vi "Post-Install Custom Action.vi"(10 "Variant":variant) -> (0 "error out":errorcluster)   [LabVIEW 2014]
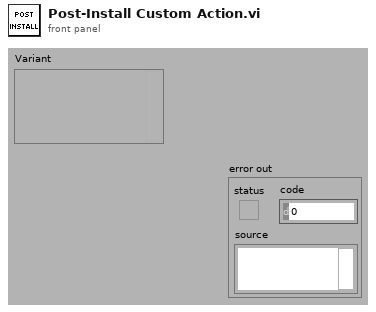
[diagram p1: front panel]
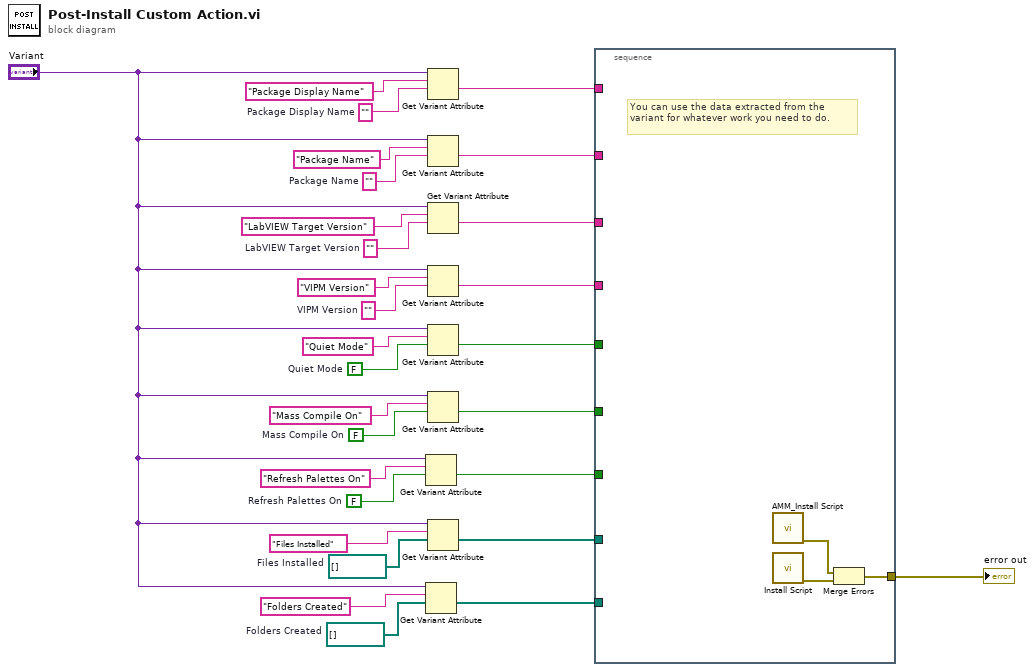
[diagram p0: block diagram]
diagram:
  w2 = path[] []  # Folders Created
  w3 = path[] []  # Files Installed
  w9 = FALSE  # Refresh Palettes On
  w10 = FALSE  # Mass Compile On
  w13 = ""  # Package Display Name
  w20 = FALSE  # Quiet Mode
  w23 = ""  # VIPM Version
  w25 = ""  # LabVIEW Target Version
  w27 = ""  # Package Name
  n1 = Get Variant Attribute(Variant="Variant", name="Refresh Palettes On", default value (empty Variant)=w9) -> (value=w12:bool)  [unwired: 1 in, 3 out]
  n2 = Get Variant Attribute(Variant="Variant", name="Folders Created", default value (empty Variant)=w2) -> (value=w7:path[])  [unwired: 1 in, 3 out]
  n3 = Get Variant Attribute(Variant="Variant", name="Package Display Name", default value (empty Variant)=w13) -> (value=w19:string)  [unwired: 1 in, 3 out]
  n4 = Get Variant Attribute(Variant="Variant", name="Package Name", default value (empty Variant)=w27) -> (value=w18:string)  [unwired: 1 in, 3 out]
  n5 = Get Variant Attribute(Variant="Variant", name="LabVIEW Target Version", default value (empty Variant)=w25) -> (value=w17:string)  [unwired: 1 in, 3 out]
  n6 = Get Variant Attribute(Variant="Variant", name="VIPM Version", default value (empty Variant)=w23) -> (value=w16:string)  [unwired: 1 in, 3 out]
  n7 = Get Variant Attribute(Variant="Variant", name="Quiet Mode", default value (empty Variant)=w20) -> (value=w15:bool)  [unwired: 1 in, 3 out]
  n8 = Get Variant Attribute(Variant="Variant", name="Mass Compile On", default value (empty Variant)=w10) -> (value=w14:bool)  [unwired: 1 in, 3 out]
  n9 = Get Variant Attribute(Variant="Variant", name="Files Installed", default value (empty Variant)=w3) -> (value=w6:path[])  [unwired: 1 in, 3 out]
  n10 = stacked-sequence {
    tunnel: w19 -> [_]
    tunnel: w18 -> [_]
    tunnel: w17 -> [_]
    tunnel: w16 -> [_]
    tunnel: w15 -> [_]
    tunnel: w14 -> [_]
    tunnel: w12 -> [_]
    tunnel: w6 -> [_]
    tunnel: w7 -> [_]
    tunnel: [w30] -> w1
    frame #0 {
      # "You can use the data extracted from the variant for whatever work you need to do."
      n11 = call "AMM_Install Script.vi"() -> ("error out"=w31:errorcluster)  [unwired: 11 in]
      n12 = call "Install Script.vi"() -> ("error out"=w32:errorcluster)  [unwired: 11 in]
      n13 = Merge Errors(w31, w32) -> (w30:errorcluster)
    }
  }
  "error out" <- w1
